vi "Predictie.vi"() -> ()   [LabVIEW 2024]
uses:
  <vilib>/National Instruments/NI Super Simple Neural Networks/Neural Network.lvclass
panel:
  in  "Training Path":path
  in  "Ora [h]":dbl(slide) scale=0.0..24.0
  in  "Radiatia Solara [W/m²]":dbl(slide) scale=0.0..1000.0
  in  "Viteza Vantului [m/s]":dbl(slide) scale=0.0..20.0
  in  "Temperatura [°C]":dbl(slide) scale=0.0..50.0
  out "2D Picture":picture
  out "Acoperire Nori [%]":dbl format="%#.2f"
  in  "Image Path":path
  in  "Stop":bool
  out "Productie [W]":dbl format="%#.2f"
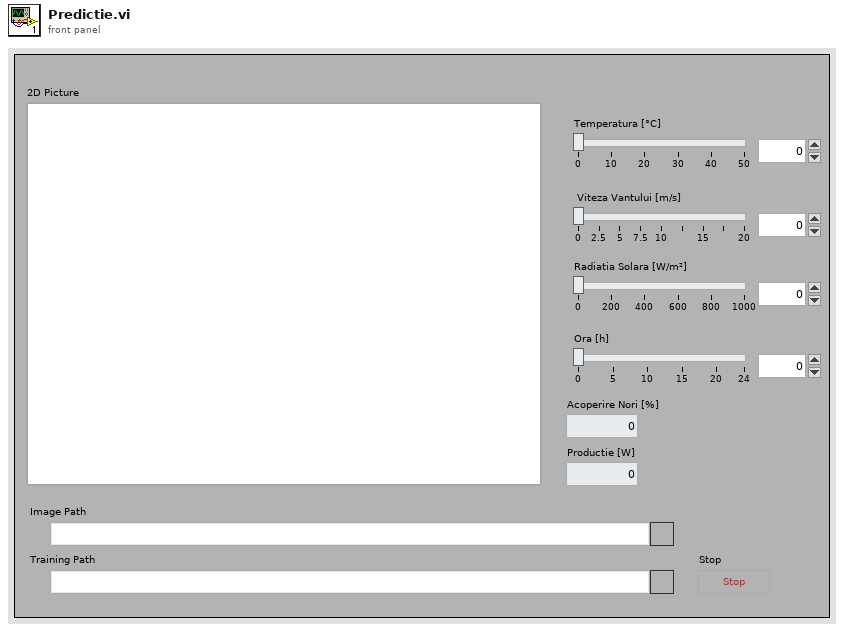
[diagram p1: front panel]
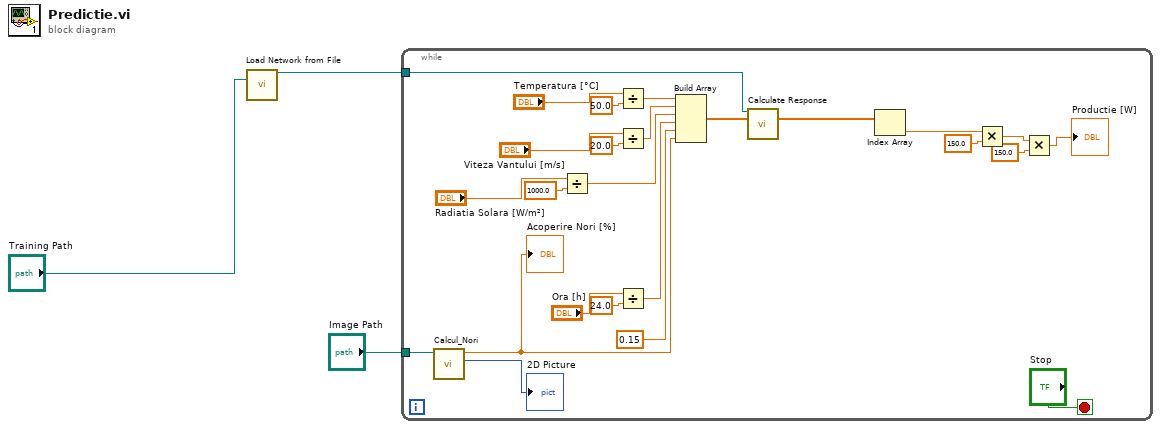
[diagram p0: block diagram]
diagram:
  n1 = call <vilib>:"Load Network from File.vi"("File Path (dialog)"="Training Path") -> ("Neural Network Out"=w3:refnum<class "Neural Network.lvclass">)  [unwired: 11 in, 3 out]
  n2 = while {
    tunnel: w3 -> [w27]
    tunnel: "Image Path" -> [w25]
    stop <- "Stop" stop-if-true
    n3 = call "Calcul_Nori.vi"("Cale Imagine"=w25) -> ("2D Picture"=→"2D Picture":picture, "Procent Nori"=w21:dbl)  [unwired: 9 in]
    "Acoperire Nori [%]" <- w21
    n4 = Divide(x="Radiatia Solara [W/m²]", y=1000.0) -> (x/y=w9:dbl)
    n5 = Divide(x="Temperatura [°C]", y=50.0) -> (x/y=w11:dbl)
    n6 = Divide(x="Viteza Vantului [m/s]", y=20.0) -> (x/y=w10:dbl)
    n7 = Divide(x="Ora [h]", y=24.0) -> (x/y=w8:dbl)
    n8 = Build Array "Build Array"(w11, w10, w9, w8, 0.15, w21) -> (w7:dbl[])
    n9 = call <vilib>:"Calculate Response.vi"("Neural Network In"=w27, "Inputs"=w7) -> ("Outputs"=w26:dbl[])  [unwired: 11 in, 2 out]
    n10 = Index Array "Index Array"(array=w26) -> (element=w23:dbl)  [unwired: 1 in]
    n11 = Multiply(x=w23, y=150.0) -> (x*y=w5:dbl)
    n12 = Multiply(x=w5, y=150.0) -> (x*y=→"Productie [W]":dbl)
  }
